vi "Advance Settings UI.vi"(0 "Advance Setting":T2, 11 "error in (no error)":errorcluster) -> (4 "Advance Setting Out":T2, 15 "error out":errorcluster)   [LabVIEW 2020, in "LDO Load Regulation.lvlib"]
uses:
  LDO Load Regulation.lvlib
  Typedefs/Advance Settings.ctl
  Typedefs/Adv Setup.ctl
  Reusables/Instrument APIs/Load Output Function.ctl
  Typedefs/Adv StimulusMeasure.ctl
  <userlib>/_Soliton/Measurement Suite/Reusables/Queue Driver/Plugin Queue Driver.lvlib
  <userlib>/_Soliton/Measurement Suite/Reusables/Plugin Common/Plugin Common.lvlib
panel:
  in  "Output Function":T1
  in  "Close":bool
  in  "Loop Delay (ms)":u32 caption="Delay between Stimulus and Measure (ms)"
  in  "Panel Close":bool
  out "Banner":picture caption="Advance Settings"
  # "For Each Current Sweep"
  # "Load SMU"
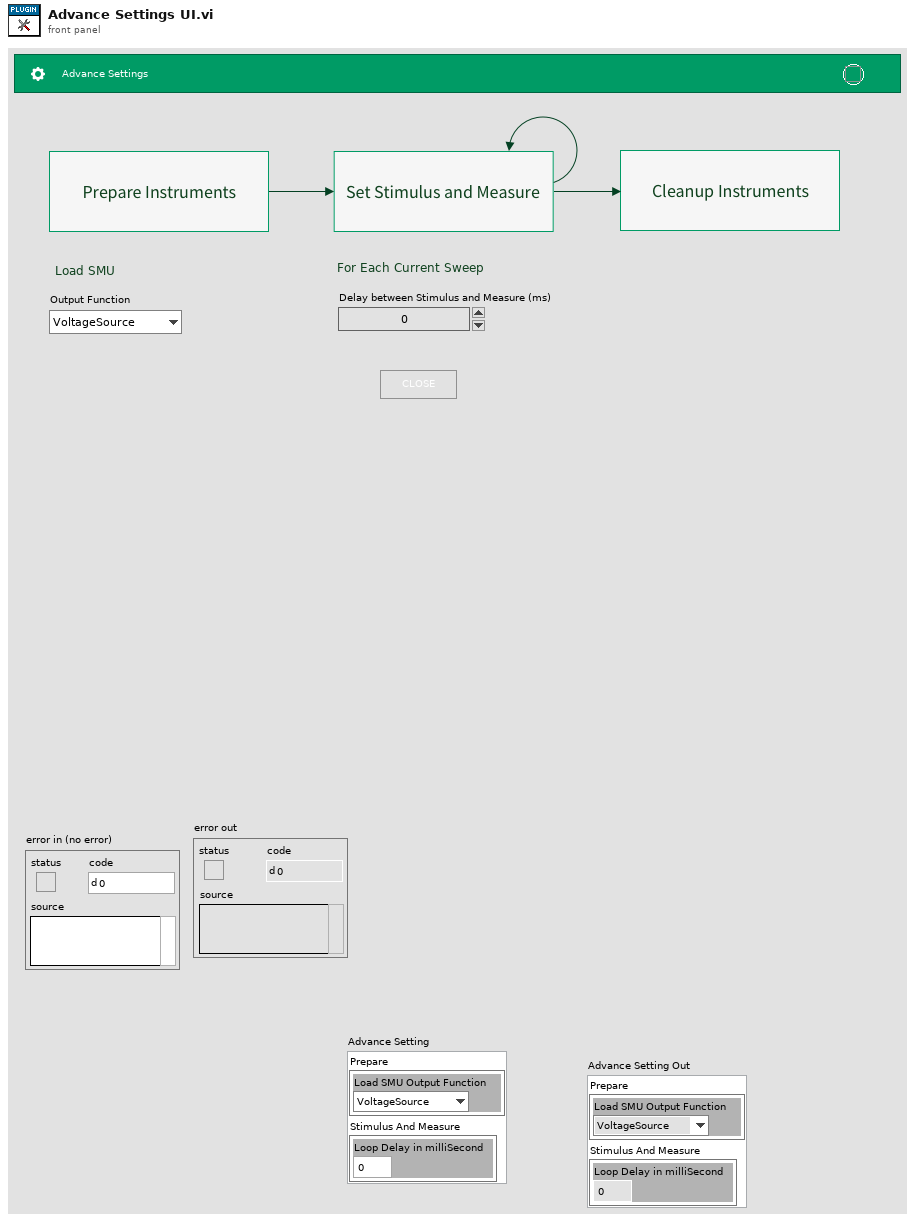
[diagram p1: front panel]
types:
  T1 = typedef "Load Output Function.ctl" = enum16{"VoltageSource", "CurrentSource"}
  T2 = typedef "LDO Load Regulation.lvlib/Advance Settings.ctl" = cluster{"Prepare":T3, "Stimulus And Measure":T4}
  T3 = typedef "LDO Load Regulation.lvlib/Adv Setup.ctl" = cluster{"Load SMU Output Function":T1}
  T4 = typedef "LDO Load Regulation.lvlib/Adv StimulusMeasure.ctl" = cluster{"Loop Delay in milliSecond":u32}
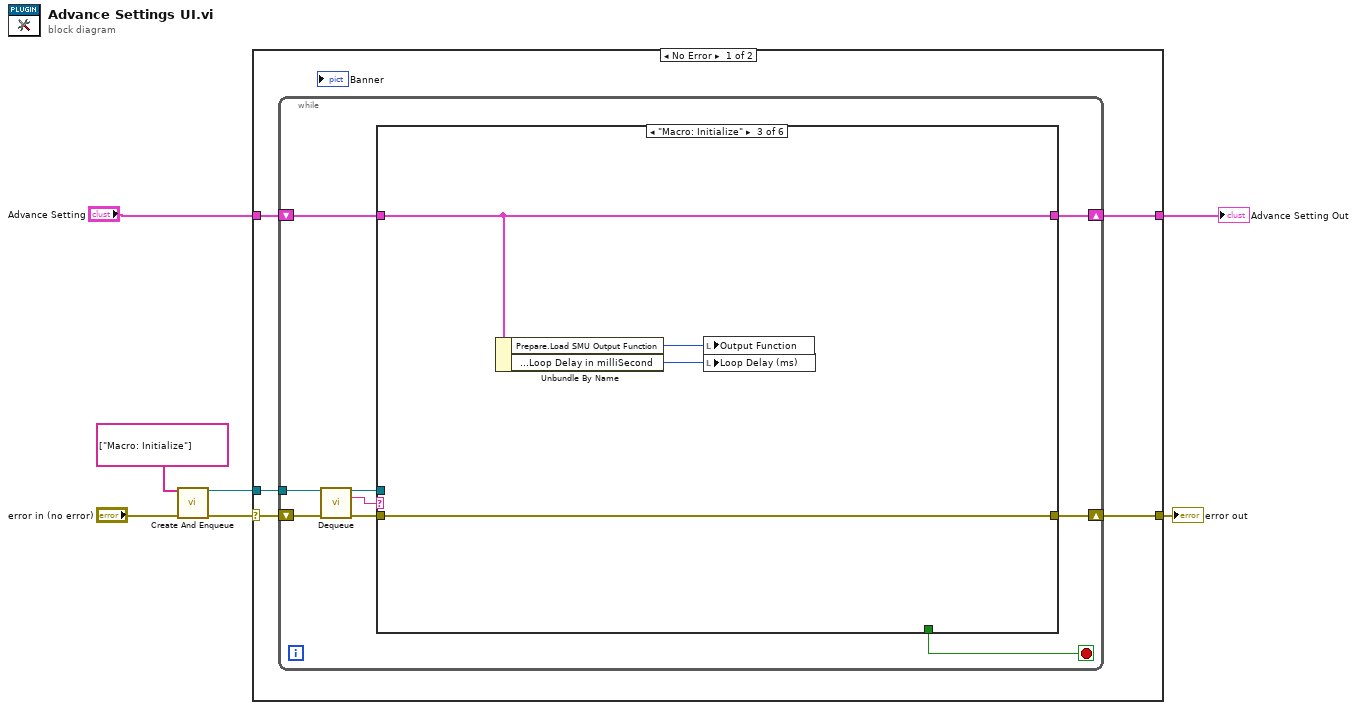
[diagram p0: block diagram]
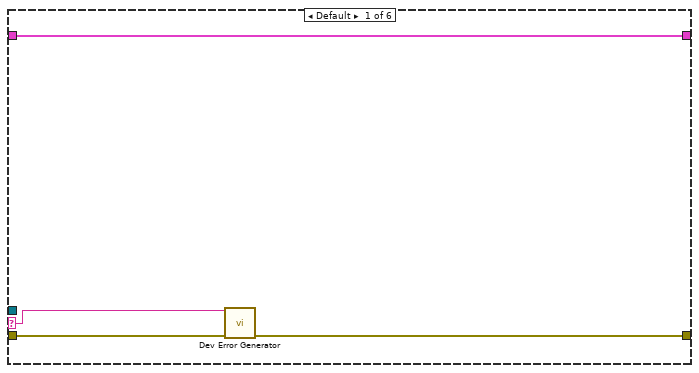
[diagram p2: hidden frame]
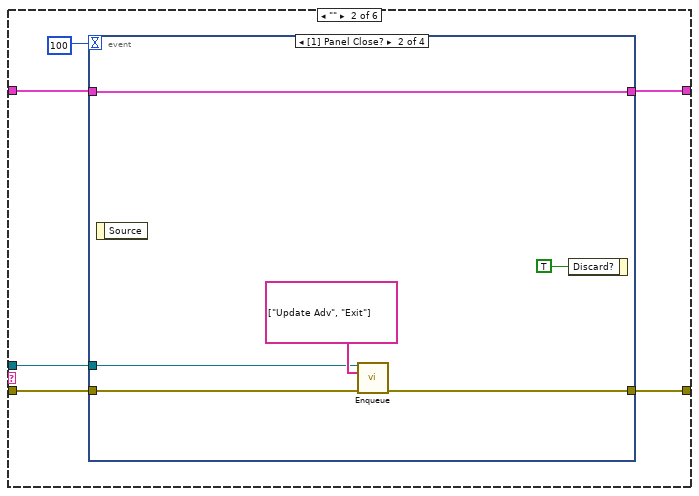
[diagram p3: hidden frame]
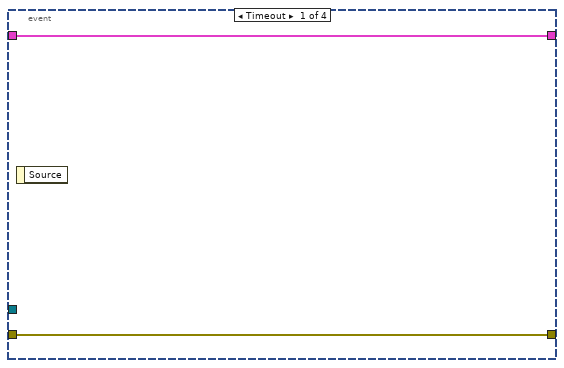
[diagram p4: hidden frame]
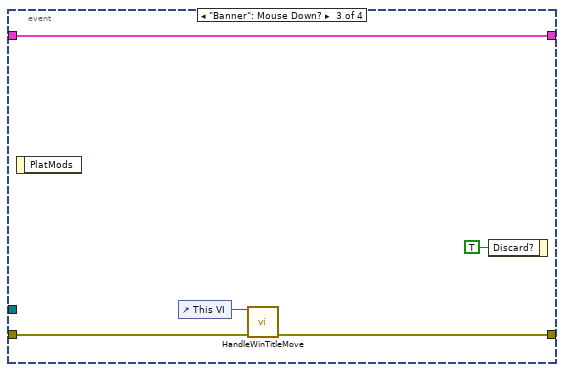
[diagram p5: hidden frame]
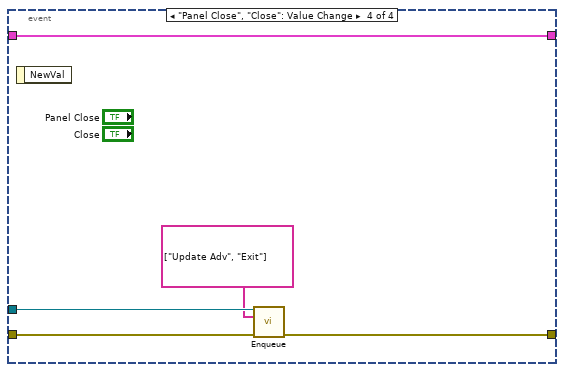
[diagram p6: hidden frame]
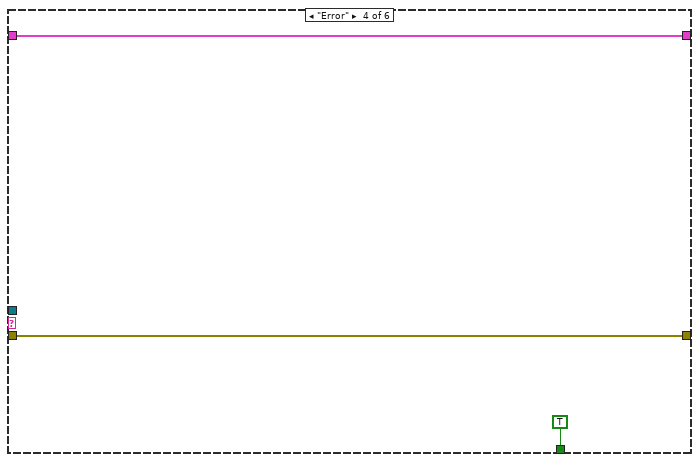
[diagram p7: hidden frame]
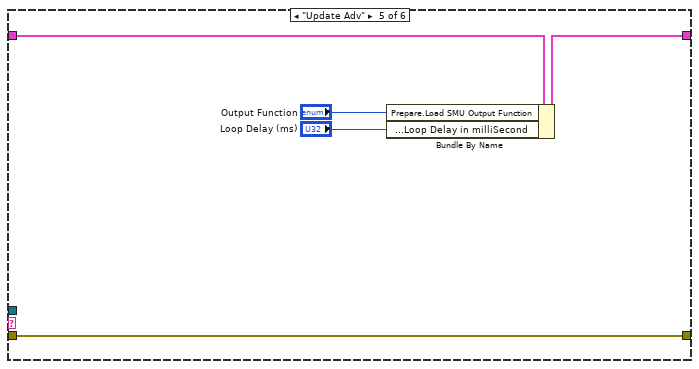
[diagram p8: hidden frame]
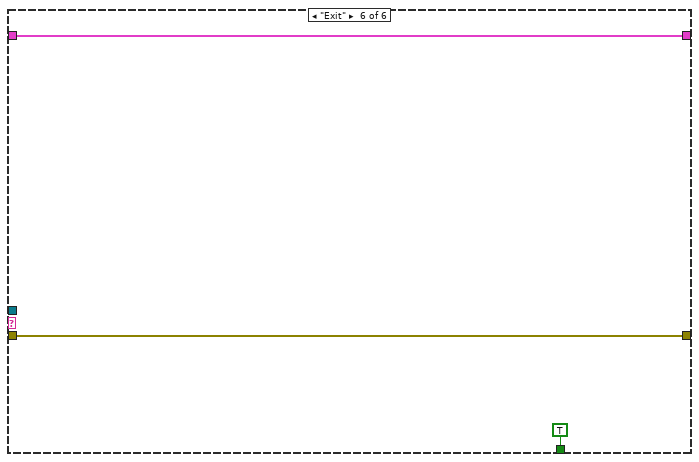
[diagram p9: hidden frame]
diagram:
  n1 = call <userlib>:"Create And Enqueue.vi"("Initial States"=string[] ["Macro: Initialize"], "error in (no error)"="error in (no error)") -> ("Queue out"=w4:refnum<queue>, "error out"=w5:errorcluster)  [unwired: 12 in]
  n2 = case shown="No Error" w5 {
    selector: w5 -> [w8 w66]
    tunnel: [w12 w66] -> w7
    tunnel: "Advance Setting" -> [w11 w65]
    tunnel: [w10 w65] -> w1
    tunnel: w4 -> [w9 _]
    frame No Error {
      n3 = while {
        tunnel: w9 -> [w18]
        shift-right: [w19] -> w10
        shift-left: w11 -> [w20]
        shift-right: [w21] -> w12
        shift-left: w8 -> [w17]
        stop <- w14 stop-if-true
        n4 = call <userlib>:"Dequeue.vi"("Queue in"=w18, "error in (no error)"=w17) -> ("Queue out"=w13:refnum<queue>, "Dequeued State"=w15:string, "error out"=w16:errorcluster)  [unwired: 11 in]
        n5 = case shown="\"Macro: Initialize\"" w15 {
          selector: w15 -> [w22 _ _ _ _ _]
          tunnel: [w24 w31 w53 w55 w61 w64] -> w21
          tunnel: w20 -> [w25 w30 w52 w56 w57 w63]
          tunnel: [w25 w29 w52 w56 w58 w63] -> w19
          tunnel: w16 -> [w23 w28 w53 w55 w61 w64]
          tunnel: [_ _ _ TRUE _ TRUE ("Discard?")] -> w14
          tunnel: w13 -> [_ w26 _ _ _ _]
          frame Default {
            n6 = call <userlib>:"Dev Error Generator.vi"("State"=w22, "error in (no error)"=w23) -> ("error out"=w24:errorcluster)  [unwired: 13 in]
          }
          frame "" {
            n7 = event shown="[1] Panel Close?" {
              selector: _ -> [_ _ _ _]
              dyn-events: _ -> [_ _ _ _]
              timeout: 100 -> [_ _ _ _]
              tunnel: w28 -> [w33 w34 w41 w47]
              tunnel: [w33 w35 w42 w48] -> w31
              tunnel: w30 -> [w32 w39 w44 w49]
              tunnel: [w32 w39 w44 w49] -> w29
              tunnel: w26 -> [_ w36 _ w46]
              event Timeout {
                n8 = event-data() -> ()  [unwired: 1 in, 1 out]
              }
              event Panel Close? {
                n9 = event-data() -> ()  [unwired: 1 in, 1 out]
                n10 = call <userlib>:"Enqueue.vi"("Queue in"=w36, "States"=string[] ["Update Adv", "Exit"] ("Initial States"), "error in (no error)"=w34) -> ("error out"=w35:errorcluster)  [unwired: 11 in, 1 out]
                n11 = event-data("Discard?"=TRUE) -> ()  [unwired: 1 in, 1 out]
              }
              event "Banner": Mouse Down? {
                n12 = event-data() -> ()  [unwired: 1 in, 1 out]
                n13 = control-ref of="This VI"() -> (w40:refnum<vi>)
                n14 = call "HandleWinTitleMove.vi"("VI in"=w40, "error in (no error)"=w41) -> ("error out"=w42:errorcluster)  [unwired: 12 in, 1 out]
                n15 = event-data("Discard?"=TRUE) -> ()  [unwired: 1 in, 1 out]
              }
              event "Panel Close", "Close": Value Change {
                n16 = event-data() -> ()  [unwired: 1 in, 1 out]
                n17 = call <userlib>:"Enqueue.vi"("Queue in"=w46, "States"=string[] ["Update Adv", "Exit"] ("Initial States"), "error in (no error)"=w47) -> ("error out"=w48:errorcluster)  [unwired: 11 in, 1 out]
              }
            }
          }
          frame "Macro: Initialize" {
            n18 = Unbundle By Name(w52) -> ("Prepare.Load SMU Output Function"=w51:T1, "Stimulus And Measure.Loop Delay in milliSecond"=w50:u32)
            n19 = local write "Output Function"(w51) -> ()
            n20 = local write "Loop Delay (ms)"(w50) -> ()
          }
          frame "Error" {
          }
          frame "Update Adv" {
            n21 = Bundle By Name(cluster=w57, "Prepare.Load SMU Output Function"="Output Function", "Stimulus And Measure.Loop Delay in milliSecond"="Loop Delay (ms)") -> (w58:T2)
          }
          frame "Exit" {
          }
        }
      }
    }
    frame Error {
    }
  }
  "error out" <- w7
  "Advance Setting Out" <- w1
